vi "SCE_calc_char_pos_offset.vi"(8 "row":i32, 9 "col":i32, 11 "VIC-II":T1) -> (3 "pos":cluster{"x":i16, "y":i16})   [LabVIEW 2018]
uses:
  SCE_VIC-II_registry.ctl
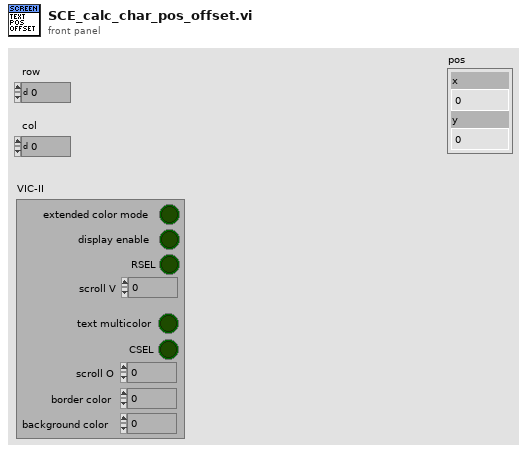
[diagram p1: front panel]
types:
  T1 = typedef "SCE_VIC-II_registry.ctl" = cluster{"extended color mode":bool, "display enable":bool, "RSEL":bool, "scroll V":u8, "text multicolor":bool, "CSEL":bool, "scroll O":u8, "border color":u8, "background color":u8}
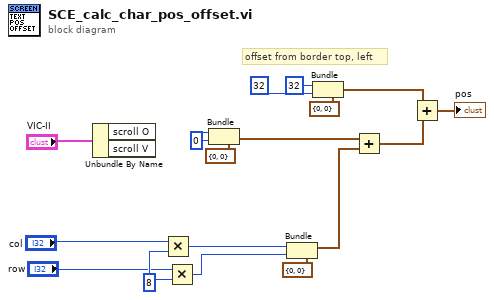
[diagram p0: block diagram]
diagram:
  w1 = i16 0 ("y")
  w11 = 8 ("y")
  # "offset from border top, left"
  n1 = Unbundle By Name("VIC-II") -> ()  [unwired: 2 out]
  n2 = Multiply(x="col", y=w11) -> (x*y=w13:i32)
  n3 = Multiply(x="row", y=w11) -> (x*y=w12:i32)
  n4 = Bundle(cluster=cluster{"x":i16, "y":i16} {"x"=0, "y"=0} ("top left point(0, 0)"), "x"=w1, "y"=w1) -> (w16:cluster{"x":i16, "y":i16})
  n5 = Bundle(cluster=cluster{"x":i16, "y":i16} {"x"=0, "y"=0} ("top left point(0, 0)"), "x"=w13, "y"=w12) -> (w8:cluster{"x":i16, "y":i16})
  n6 = Bundle(cluster=cluster{"x":i16, "y":i16} {"x"=0, "y"=0} ("top left point(0, 0)"), "x"=i16 32, "y"=i16 32 ("x")) -> (w6:cluster{"x":i16, "y":i16})
  n7 = Add(x=w16, y=w8) -> (x+y=w5:cluster{"x":i16, "y":i16})
  n8 = Add(x=w6, y=w5) -> (x+y=→"pos":cluster{"x":i16, "y":i16})
